vi "Configure Waveform Timing and PA Control.vi"(0 "RFSG handle":refnum<k15>, 5 "Waveform":T4={"Waveform Name"="Wfm", "Waveform"={"x0"=0.0, "dx"=0.0, "y"=[]}, "Signal Bandwidth (Hz)"=0.0, "PAPR (dB)"=0.0, "Burst Length (s)"=0.0, "Sample Rate"=0.0, "Burst Start Locations"=[], "Burst Stop Locations"=[], "Idle Duration Present?"=FALSE} {"Sample Rate" format="%#_6p"; "Burst Length (s)" format="%#_6p"; "PAPR (dB)" format="%.2f"; "Signal Bandwidth (Hz)" format="%.2f"; "Waveform"."y" format="%.2f"; "Waveform"."dx" format="%^.2e"; "Waveform"."x0" format="%^.2e"}, 7 "Waveform Timing Configuration":T3={"Duty Cycle (%)"=50.0, "Pre-Burst Time (s)"=1e-06, "Post-Burst Time (s)"=1e-06} {"Post-Burst Time (s)" format="%#_6p"; "Pre-Burst Time (s)" format="%#_6p"; "Duty Cycle (%)" min=1.0 max=100.0 step=1.0 format="%#_2d%%"}, 9 "PAEN Configuration":T1={"PAEN Mode"=enum."Dynamic", "Command Enable Time (s)"=0.0, "Command Disable Time (s)"=0.0, "PA Enable Trigger Mode"=23001, "PA Enable Trigger Export Terminal"="PFI0"} {"PA Enable Trigger Mode" items=["Pulse"=23000, "Toggle"=23001]; "Command Disable Time (s)" format="%#_6p"; "Command Enable Time (s)" format="%#_6p"}, 11 "error in":errorcluster) -> (4 "RFSG handle out":refnum<k15>, 6 "Generation Period (s)":dbl, 15 "error out":errorcluster)   [LabVIEW 2018, in "SG.lvlib"]
uses:
  SG.lvlib
  Typedefs/Waveform.ctl
  Typedefs/Waveform Timing Configuration.ctl
  Typedefs/PAEN Configuration.ctl
  <instrlib>/niRFSG/niRFSG.llb/niRFSG Exported Signal Destinations.ctl
  <instrlib>/niRFSG/niRFSG.llb/niRFSG Signal Names.ctl
  <instrlib>/niRFSG/niRFSG.llb/niRFSG Signal Identifiers.ctl
  <instrlib>/niRFSG/niRFSG.llb/niRFSG Script Trigger IDs.ctl
  <instrlib>/niRFSGPlayback/niRFSGPlayback Set Script to Generate (1 RFSG).vi
  <instrlib>/niRFSG/niRFSG.llb/niRFSG Configure Script Trigger Software.vi
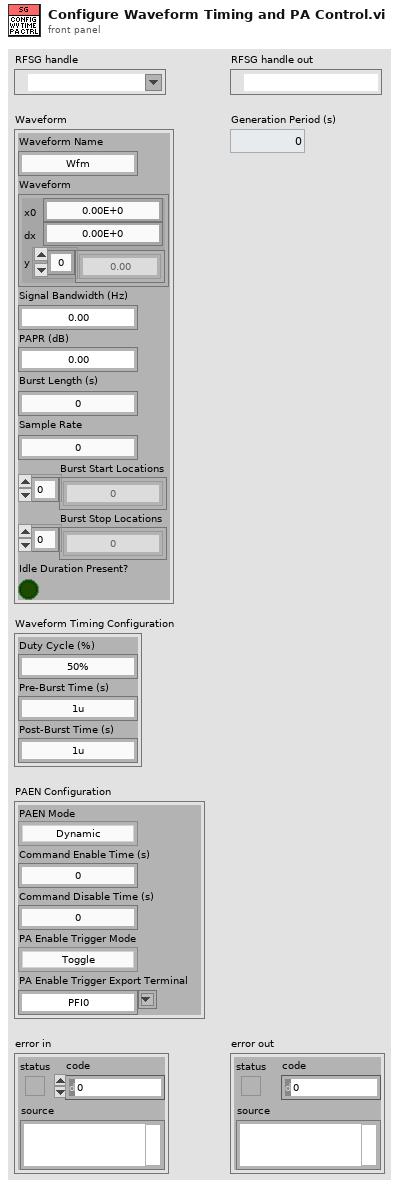
[diagram p1: front panel]
types:
  T1 = typedef "SG.lvlib/PAEN Configuration.ctl" = cluster{"PAEN Mode":enum16{"Disabled", "Static", "Dynamic"}, "Command Enable Time (s)":dbl, "Command Disable Time (s)":dbl, "PA Enable Trigger Mode":i32, "PA Enable Trigger Export Terminal":T2}
  T2 = typedef "niRFSG Exported Signal Destinations.ctl" = string
  T3 = typedef "SG.lvlib/Waveform Timing Configuration.ctl" = cluster{"Duty Cycle (%)":dbl, "Pre-Burst Time (s)":dbl, "Post-Burst Time (s)":dbl}
  T4 = typedef "SG.lvlib/Waveform.ctl" = cluster{"Waveform Name":string, "Waveform":cluster{"x0":dbl, "dx":dbl, "y":csg[]}, "Signal Bandwidth (Hz)":dbl, "PAPR (dB)":dbl, "Burst Length (s)":dbl, "Sample Rate":dbl, "Burst Start Locations":i32[], "Burst Stop Locations":i32[], "Idle Duration Present?":bool}
  T5 = typedef "niRFSG Script Trigger IDs.ctl" = string
  T6 = typedef "niRFSG Signal Identifiers.ctl" = string
  T7 = typedef "niRFSG Signal Names.ctl" = i32
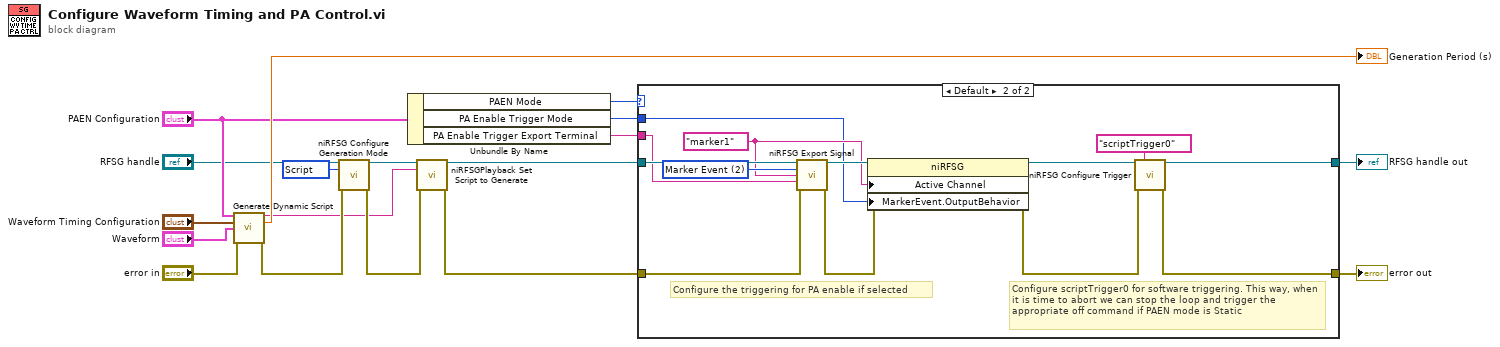
[diagram p0: block diagram]
diagram:
  w1 = 1002 items=["CW"=1000, "Arb Waveform"=1001, "Script"=1002] ("generation mode")
  n1 = call "Generate Dynamic Script.vi"("PAEN Config"="PAEN Configuration", "Waveform Timing Configuration"="Waveform Timing Configuration", "Waveform"="Waveform", "error in (no error)"="error in") -> ("Script"=w2:string, "Generation Period (s)"=→"Generation Period (s)":dbl, "error out"=w4:errorcluster)  [unwired: 9 in]
  n2 = call <instrlib>:"niRFSG Configure Generation Mode.vi"("instrument handle"="RFSG handle", "generation mode"=w1, "error in"=w4) -> ("instrument handle out"=w5:refnum<k15>, "error out"=w3:errorcluster)  [unwired: 11 in]
  n3 = Unbundle By Name("PAEN Configuration") -> ("PAEN Mode"=w13:enum16{"Disabled", "Static", "Dynamic"}, "PA Enable Trigger Mode"=w9:i32, "PA Enable Trigger Export Terminal"=w6:T2)
  n4 = call-poly <instrlib>:"niRFSGPlayback Set Script to Generate.vi"("instrument handle in"=w5, "script text"=w2, "error in"=w3) -> ("instrument handle out"=w10:refnum<k15>, "error out"=w7:errorcluster)  [unwired: 11 in]
  n5 = case "Configure the triggering for PA enable if selected" shown="Default" w13 {
    tunnel: [w20 w21] -> w12
    tunnel: w7 -> [w20 w30]
    tunnel: [w19 w23] -> w11
    tunnel: w10 -> [w19 w33]
    tunnel: w9 -> [_ w27]
    tunnel: w6 -> [_ w25]
    frame "Disabled" {
    }
    frame Default {
      w28 = T6 "marker1" ("signal identifier")
      w31 = T7 2 items=["Start Trigger", "Script Trigger", "Marker Event", "Ref Clock", "Started Event", "Done Event", "Configuration List Step Trigger", "Configuration Settled Event"] ("signal")
      # "Configure the triggering for PA enable if selected"
      # "Configure scriptTrigger0 for software triggering. This way, when it is time to abort we can stop the loop and trigger the appropriate off command if PAEN mode is Static"
      n6 = call <instrlib>:"niRFSG Export Signal.vi"("instrument handle"=w33, "signal"=w31, "signal identifier"=w28, "output terminal"=w25, "error in"=w30) -> ("instrument handle out"=w32:refnum<k15>, "error out"=w29:errorcluster)  [unwired: 9 in]
      n7 = property class="niRFSG"(reference=w32, error in=w29, "Active Channel"=w28, "MarkerEvent.OutputBehavior"=w27) -> (reference out=w24:refnum<k15>, error out=w26:errorcluster)
      n8 = call-poly <instrlib>:"niRFSG Configure Trigger.vi"("instrument handle"=w24, "trigger id"=T5 "scriptTrigger0", "error in"=w26) -> ("instrument handle out"=w23:refnum<k15>, "error out"=w21:errorcluster)  [unwired: 11 in]
    }
  }
  "RFSG handle out" <- w11
  "error out" <- w12
